vi "JoyStick_Deadband.vi"(2 "DeadbandY":dbl, 3 "DeadbandX":dbl, 4 "Y":dbl, 5 "X":dbl) -> (0 "OutY":dbl, 1 "OutX":dbl)   [LabVIEW 2014]
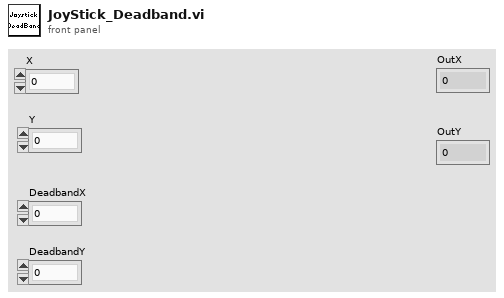
[diagram p1: front panel]
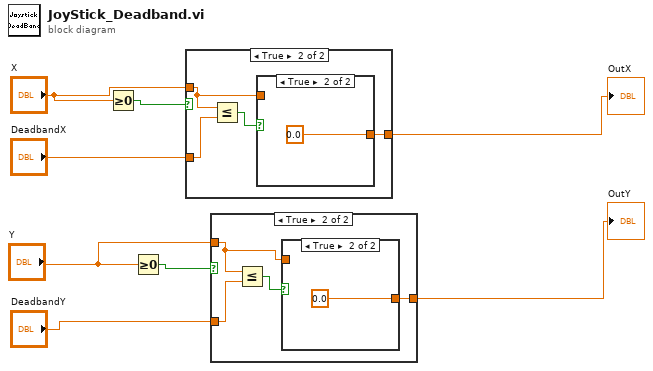
[diagram p0: block diagram]
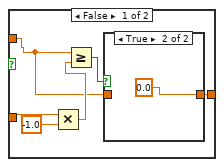
[diagram p2: hidden frame]
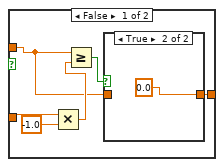
[diagram p5: hidden frame]
diagram:
  n1 = Greater Or Equal To 0?(x="X") -> (x >= 0?=w8:bool)
  n2 = Greater Or Equal To 0?(x="Y") -> (x >= 0?=w4:bool)
  n3 = case shown="True" w8 {
    tunnel: "DeadbandX" -> [w14 w20]
    tunnel: "X" -> [w9 w17]
    tunnel: [w10 w18] -> w5
    frame False {
      n4 = Multiply(x=w14, y=-1.0) -> (x*y=w12:dbl)
      n5 = Greater Or Equal?(x=w9, y=w12) -> (x >= y?=w11:bool)
      n6 = case shown="True" w11 {
        tunnel: [w15 0.0] -> w10
        tunnel: w9 -> [w15 _]
        frame False {
        }
        frame True {
        }
      }
    }
    frame True {
      n7 = Less Or Equal?(x=w17, y=w20) -> (x <= y?=w19:bool)
      n8 = case shown="True" w19 {
        tunnel: [w21 0.0] -> w18
        tunnel: w17 -> [w21 _]
        frame False {
        }
        frame True {
        }
      }
    }
  }
  "OutX" <- w5
  n9 = case shown="True" w4 {
    tunnel: "DeadbandY" -> [w28 w34]
    tunnel: [w24 w32] -> w1
    tunnel: "Y" -> [w23 w31]
    frame False {
      n10 = Multiply(x=w28, y=-1.0) -> (x*y=w26:dbl)
      n11 = Greater Or Equal?(x=w23, y=w26) -> (x >= y?=w25:bool)
      n12 = case shown="True" w25 {
        tunnel: [w29 0.0] -> w24
        tunnel: w23 -> [w29 _]
        frame False {
        }
        frame True {
        }
      }
    }
    frame True {
      n13 = Less Or Equal?(x=w31, y=w34) -> (x <= y?=w33:bool)
      n14 = case shown="True" w33 {
        tunnel: [w35 0.0] -> w32
        tunnel: w31 -> [w35 _]
        frame False {
        }
        frame True {
        }
      }
    }
  }
  "OutY" <- w1
